vi "Test_ReadItem_WrongType_Error.vi"(8 "error in (no error)":errorcluster, 11 "TestCase in":refnum<class "TestComposedLookupTable.lvclass">) -> (0 "error out":errorcluster, 3 "TestCase out":refnum<class "TestComposedLookupTable.lvclass">)   [LabVIEW 2017, in "TestComposedLookupTable.lvclass"]
uses:
  TestComposedLookupTable.lvclass
  Source/LookupTable/LookupTable.lvclass/LookupTable.ctl
  eaf38a46-e02b-48d4-82be-b08a20dd1172.vi
  671f435e-2646-4ca5-ac73-9aa6e65d8a54.vi
  Source/LookupTable/Read Table Reference.vi
  eaf38a46-e02b-48d4-82be-b08a20dd1172.vi/498b67b9-71ab-4b51-990d-013cdb7264ab.vi
  671f435e-2646-4ca5-ac73-9aa6e65d8a54.vi/4de7411d-e9b5-47ea-99f0-d9e29fd168ad.vi
  Source/LookupTable/LookupTable.lvclass
panel:
  out "Return Error":errorcluster
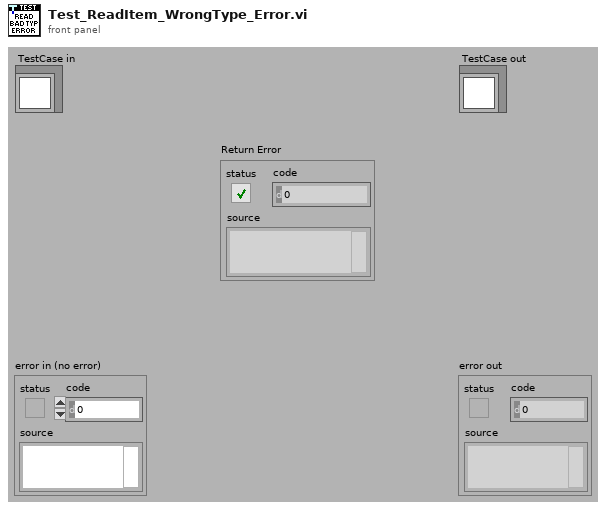
[diagram p1: front panel]
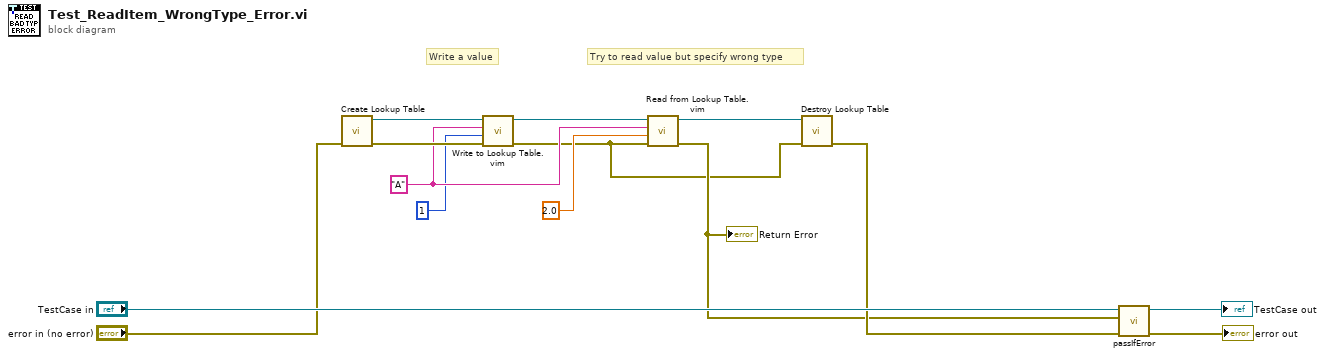
[diagram p0: block diagram]
diagram:
  w9 = "A" ("Item Name")
  # "Try to read value but specify wrong type"
  # "Write a value"
  n1 = call "Create Lookup Table.vi"("error in (no error)"="error in (no error)") -> ("error out"=w14:errorcluster, "LookupTable Reference"=w8:refnum<data-value>)  [unwired: 9 in]
  n2 = call "Write to Lookup Table.vim"("error in (no error)"=w14, "Item"=1, "Item Name"=w9, "LookupTable Reference"=w8) -> ("error out"=w1:errorcluster, "LookupTable Reference Out"=w10:refnum<data-value>)  [unwired: 5 in, 1 out]
  n3 = call "Read from Lookup Table.vim"("error in (no error)"=w1, "Type"=2.0, "Item Name"=w9, "LookupTable Reference"=w10) -> ("error out"=w2:errorcluster, "LookupTable Reference Out"=w6:refnum<data-value>)  [unwired: 4 in, 2 out]
  "Return Error" <- w2
  n4 = call "Destroy Lookup Table.vi"("error in (no error)"=w1, "LookupTable Reference"=w6) -> ("error out"=w5:errorcluster)  [unwired: 9 in]
  n5 = call-dynamic "passIfError.vi"("error in (no error)"=w5, "error"=w2, "TestCase in"="TestCase in") -> ("error out"=→"error out":errorcluster, "TestCase out"=→"TestCase out":refnum<class "TestComposedLookupTable.lvclass">)  [unwired: 7 in]
